vi "LabVIEW VI to Flatten XML.vi"(9 "Serialize VI":bool, 10 "output file":path, 11 "VI Path":path) -> (0 "error out":errorcluster, 3 "__return":string)   [LabVIEW 2014]
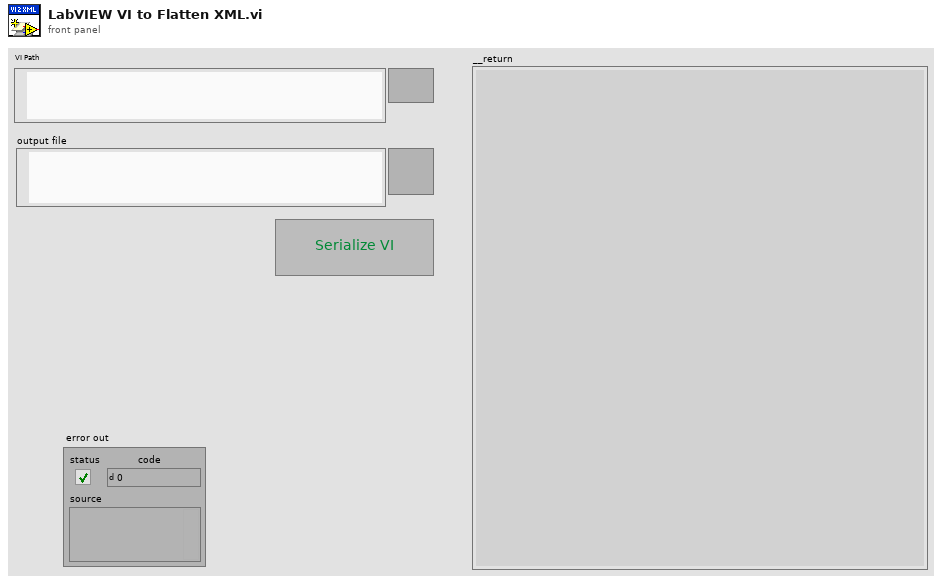
[diagram p1: front panel]
types:
  T1 = enum16{"open", "replace", "create", "open or create", "replace or create", "replace or create with confirmation"}
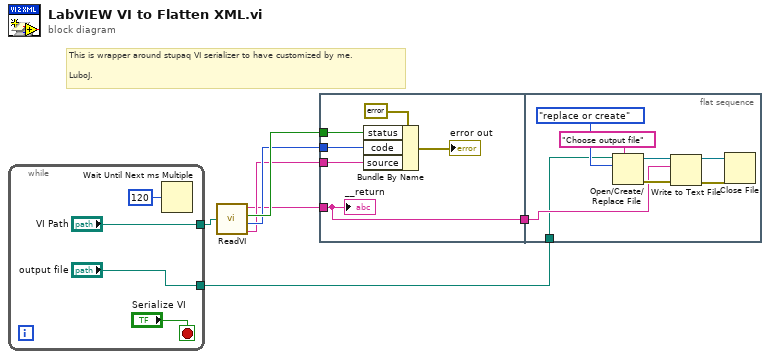
[diagram p0: block diagram]
diagram:
  # "This is wrapper around stupaq VI serializer to have customized by me.\n\nLuboJ."
  n1 = while {
    tunnel: ["output file"] -> w1
    tunnel: ["VI Path"] -> w3
    stop <- "Serialize VI" stop-if-true
    n2 = Wait Until Next ms Multiple(millisecond multiple=u32 120) -> ()  [unwired: 1 out]
  }
  n3 = call "ReadVI.vi"("VI Path"=w3) -> ("__return"=w4:string, "__errStatus"=w7:bool, "__errCode"=w6:i32, "__errSource"=w5:string)
  n4 = flat-sequence {
    tunnel: w7 -> [w13]
    tunnel: w6 -> [w14]
    tunnel: w5 -> [w15]
    tunnel: w4 -> [w17]
    tunnel: [w17] -> w2
    tunnel: w2 -> [w19]
    tunnel: w1 -> [w18]
    frame #0 {
      n5 = Bundle By Name(cluster=errorcluster {"status"=FALSE, "code"=0, "source"=""} ("error constant"), "status"=w13, "code"=w14, "source"=w15) -> (→"error out":errorcluster)
      "__return" <- w17
    }
    frame #1 {
      n6 = Open/Create/Replace File(file path (use dialog)=w18, prompt="Choose output file", operation (0:open)=T1."replace or create") -> (refnum out=w22:refnum<file>, error out=w21:errorcluster)  [unwired: 3 in, 1 out]
      n7 = Write to Text File(file (use dialog)=w22, text=w19, error in=w21) -> (refnum out=w24:refnum<file>, error out=w23:errorcluster)  [unwired: 1 in, 1 out]
      n8 = Close File(refnum=w24, error in=w23) -> ()  [unwired: 2 out]
    }
  }
